vi "DWE Read Directory.vi"(11 "path":path) -> (3 "Laundry.NET \nfile paths 3":T1)   [LabVIEW 2014]
doc: "Open folder where Boardx.csv files are stored and pull out Boardx.csv file paths to use."
panel:
  in  "Laundry.NET \nfile paths 2":T1
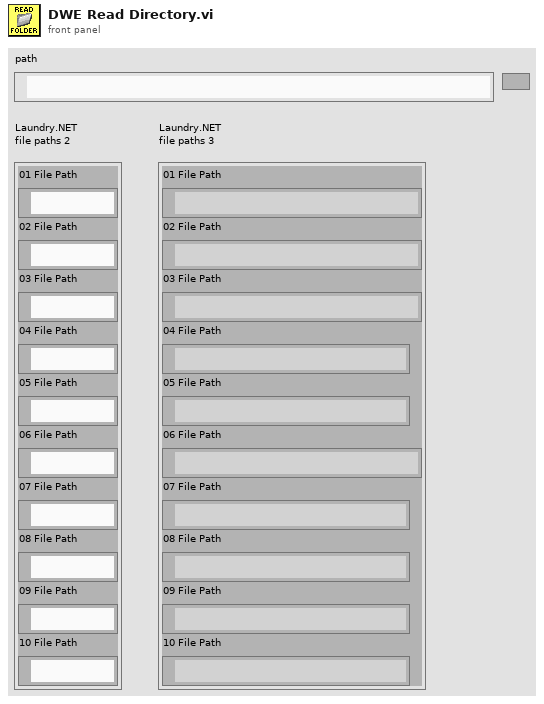
[diagram p1: front panel]
types:
  T1 = cluster{"01 File Path":path, "02 File Path":path, "03 File Path":path, "04 File Path":path, "05 File Path":path, "06 File Path":path, "07 File Path":path, "08 File Path":path, "09 File Path":path, "10 File Path":path}
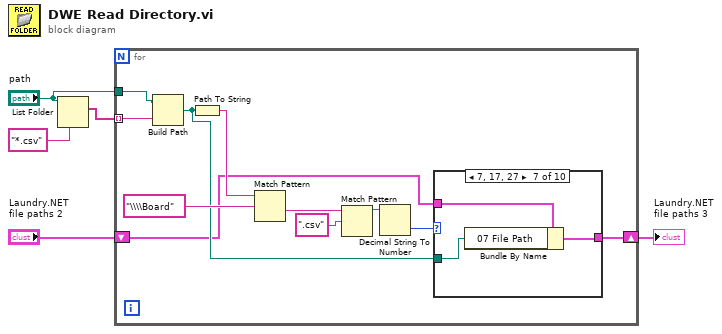
[diagram p0: block diagram]
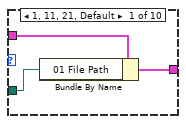
[diagram p2: hidden frame]
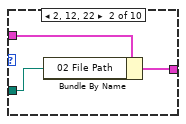
[diagram p3: hidden frame]
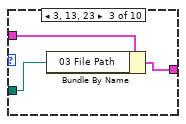
[diagram p4: hidden frame]
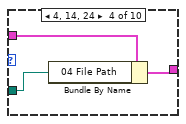
[diagram p5: hidden frame]
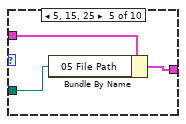
[diagram p6: hidden frame]
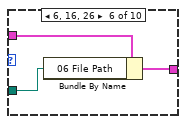
[diagram p7: hidden frame]
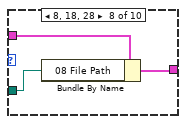
[diagram p8: hidden frame]
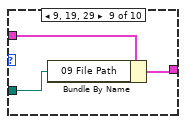
[diagram p9: hidden frame]
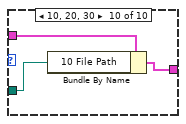
[diagram p10: hidden frame]
diagram:
  n1 = List Folder(path="path", pattern="*.csv") -> (filenames=w3:string[])  [unwired: 2 in, 3 out]
  n2 = for {
    tunnel: "path" -> [w16]
    tunnel: w3 -> [w15] mode=indexing
    shift-right: [w7] -> w2
    shift-left: "Laundry.NET \nfile paths 2" -> [w6]
    n3 = Build Path(base path=w16, name or relative path=w15) -> (appended path=w8:path)
    n4 = Path To String(path=w8) -> (string=w11:string)
    n5 = Match Pattern(string=w11, regular expression="\\\\Board") -> (after substring=w14:string)  [unwired: 1 in, 3 out]
    n6 = Match Pattern(string=w14, regular expression=".csv") -> (before substring=w10:string)  [unwired: 1 in, 3 out]
    n7 = Decimal String To Number(string=w10) -> (number=w9:i32)  [unwired: 2 in, 1 out]
    n8 = case shown="7, 17, 27" w9 {
      tunnel: w6 -> [w19 w22 w25 w28 w31 w33 w36 w40 w43 w46]
      tunnel: w8 -> [w18 w21 w24 w27 w29 w32 w35 w39 w41 w44]
      tunnel: [w17 w20 w23 w26 w30 w34 w37 w38 w42 w45] -> w7
      frame 1, 11, 21, Default {
        n9 = Bundle By Name(cluster=w19, "01 File Path"=w18) -> (w17:T1)
      }
      frame 2, 12, 22 {
        n10 = Bundle By Name(cluster=w22, "02 File Path"=w21) -> (w20:T1)
      }
      frame 3, 13, 23 {
        n11 = Bundle By Name(cluster=w25, "03 File Path"=w24) -> (w23:T1)
      }
      frame 4, 14, 24 {
        n12 = Bundle By Name(cluster=w28, "04 File Path"=w27) -> (w26:T1)
      }
      frame 5, 15, 25 {
        n13 = Bundle By Name(cluster=w31, "05 File Path"=w29) -> (w30:T1)
      }
      frame 6, 16, 26 {
        n14 = Bundle By Name(cluster=w33, "06 File Path"=w32) -> (w34:T1)
      }
      frame 7, 17, 27 {
        n15 = Bundle By Name(cluster=w36, "07 File Path"=w35) -> (w37:T1)
      }
      frame 8, 18, 28 {
        n16 = Bundle By Name(cluster=w40, "08 File Path"=w39) -> (w38:T1)
      }
      frame 9, 19, 29 {
        n17 = Bundle By Name(cluster=w43, "09 File Path"=w41) -> (w42:T1)
      }
      frame 10, 20, 30 {
        n18 = Bundle By Name(cluster=w46, "10 File Path"=w44) -> (w45:T1)
      }
    }
  }
  "Laundry.NET \nfile paths 3" <- w2
